vi "Read initial setup.vi"(8 "error in (no error)":errorcluster, 10 "use cong file":bool, 11 "Channel in":refnum<class "SPARC4_Channel.lvclass">) -> (0 "error out":errorcluster, 3 "Channel out":refnum<class "SPARC4_Channel.lvclass">)   [LabVIEW 2018, in "SPARC4_Channel.lvclass"]
uses:
  SPARC4_Channel.lvclass
  SPARC4_Channel.lvclass/SPARC4_Channel.ctl
  <vilib>/Utility/config.llb/Read Key (U32).vi
  <vilib>/Utility/config.llb/Read Key (String).vi
  <vilib>/Utility/config.llb/NI_LVConfig.lvlib
panel:
  out "Configuration to initialize ACS":T1
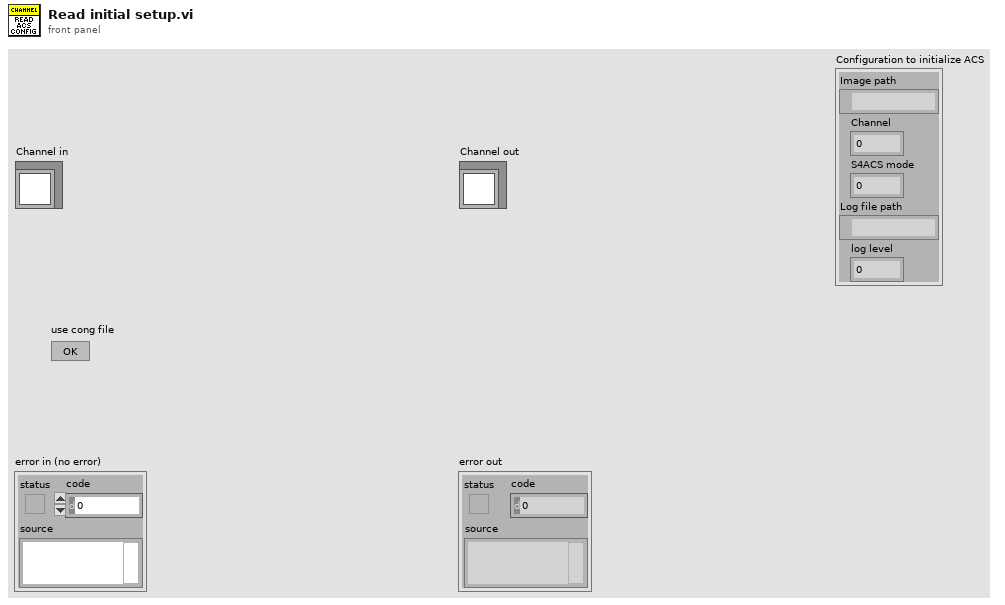
[diagram p1: front panel]
types:
  T1 = cluster{"Image path":path, "Channel":u8, "S4ACS mode":u16, "Log file path":path, "log level":u16}
  T2 = typedef "NI_LVConfig.lvlib/Config Data RefNum.ctl" = refnum<k1>
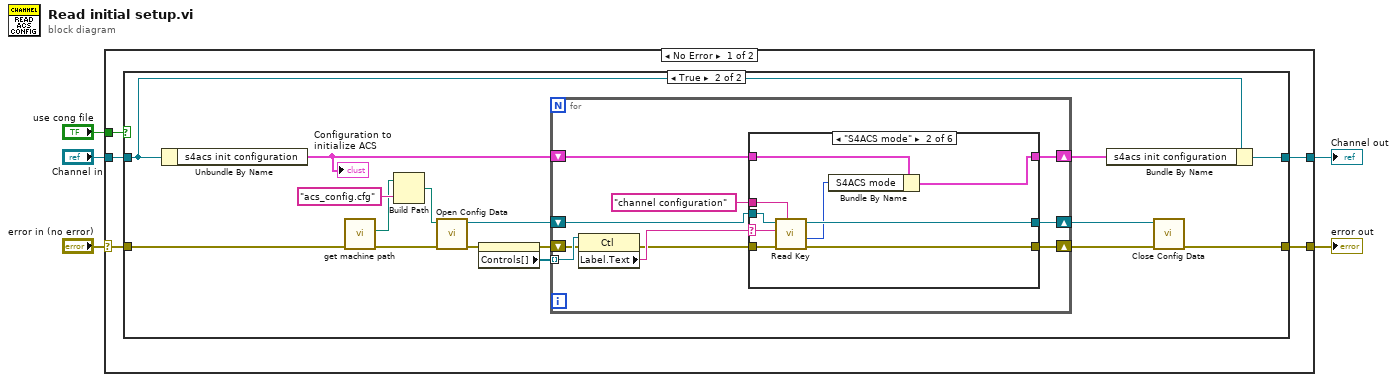
[diagram p0: block diagram]
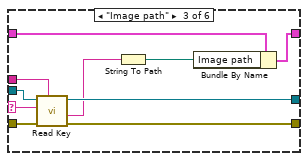
[diagram p4: hidden frame]
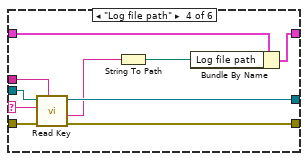
[diagram p5: hidden frame]
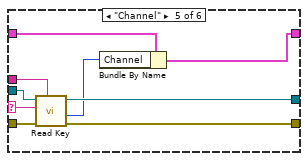
[diagram p6: hidden frame]
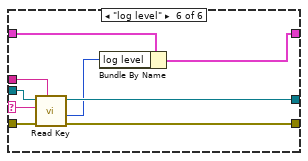
[diagram p7: hidden frame]
diagram:
  n1 = case shown="No Error" "error in (no error)" {
    selector: "error in (no error)" -> [w7 w90]
    tunnel: [w10 w90] -> w3
    tunnel: [w8 w89] -> w2
    tunnel: "Channel in" -> [w9 w89]
    tunnel: "use cong file" -> [w6 _]
    frame No Error {
      n2 = case shown="True" w6 {
        tunnel: [w11 w25] -> w10
        tunnel: w9 -> [w12 w24]
        tunnel: [w12 w22] -> w8
        tunnel: w7 -> [w11 w18]
        frame False {
        }
        frame True {
          n3 = Unbundle By Name(w24) -> ("s4acs init configuration"=w16:T1)
          "Configuration to initialize ACS" <- w16
          n4 = call "get machine path.vi"("error in (no error) 2"=w18) -> ("error in (no error)"=w19:errorcluster, "machine path"=w17:path)  [unwired: 9 in]
          n5 = Build Path(base path=w17, name or relative path="acs_config.cfg") -> (appended path=w21:path)
          n6 = call <vilib>:"Open Config Data.vi"("error in (no error)"=w19, "configuration file path"=w21) -> ("error out"=w13:errorcluster, "refnum"=w27:T2)  [unwired: 7 in, 1 out]
          n7 = property on="Configuration to initialize ACS" class="Clust (strict)"(error in=w13) -> (error out=w14:errorcluster, "Controls[]"=w15:refnum<vi>[])  [unwired: 1 in, 1 out]
          n8 = for {
            tunnel: w15 -> [w37] mode=indexing
            shift-right: [w35] -> w28
            shift-left: w14 -> [w33]
            shift-right: [w34] -> w26
            shift-left: w27 -> [w32]
            shift-right: [w30] -> w23
            shift-left: w16 -> [w38]
            n9 = property class="Ctl"(reference=w37, error in=w33) -> (error out=w31:errorcluster, "Label.Text"=w36:string)  [unwired: 1 out]
            n10 = case shown="\"S4ACS mode\"" w36 {
              selector: w36 -> [_ w48 w58 w68 w77 w86]
              tunnel: [w40 w49 w59 w69 w78 w87] -> w34
              tunnel: [w39 w50 w60 w70 w79 w88] -> w35
              tunnel: w38 -> [w41 w46 w55 w65 w75 w84]
              tunnel: [w41 w45 w54 w64 w74 w83] -> w30
              tunnel: w32 -> [w40 w43 w52 w62 w73 w82]
              tunnel: w31 -> [w39 w42 w51 w61 w72 w81]
              tunnel: "channel configuration" -> [_ w44 w53 w63 w71 w80]
              frame "False", Default {
              }
              frame "S4ACS mode" {
                n11 = call-poly <vilib>:"Read Key.vi"("section"=w44, "error in (no error)"=w42, "key"=w48, "refnum"=w43) -> ("error out"=w50:errorcluster, "value"=w47:u32, "refnum out"=w49:T2)  [unwired: 4 in, 1 out]
                n12 = Bundle By Name(cluster=w46, "S4ACS mode"=w47) -> (w45:T1)
              }
              frame "Image path" {
                n13 = call-poly <vilib>:"Read Key.vi"("section"=w53, "error in (no error)"=w51, "key"=w58, "refnum"=w52) -> ("error out"=w60:errorcluster, "value"=w56:string, "refnum out"=w59:T2)  [unwired: 4 in, 1 out]
                n14 = String To Path(string=w56) -> (path=w57:path)
                n15 = Bundle By Name(cluster=w55, "Image path"=w57) -> (w54:T1)
              }
              frame "Log file path" {
                n16 = call-poly <vilib>:"Read Key.vi"("section"=w63, "error in (no error)"=w61, "key"=w68, "refnum"=w62) -> ("error out"=w70:errorcluster, "value"=w66:string, "refnum out"=w69:T2)  [unwired: 4 in, 1 out]
                n17 = String To Path(string=w66) -> (path=w67:path)
                n18 = Bundle By Name(cluster=w65, "Log file path"=w67) -> (w64:T1)
              }
              frame "Channel" {
                n19 = call-poly <vilib>:"Read Key.vi"("section"=w71, "error in (no error)"=w72, "key"=w77, "refnum"=w73) -> ("error out"=w79:errorcluster, "value"=w76:u32, "refnum out"=w78:T2)  [unwired: 4 in, 1 out]
                n20 = Bundle By Name(cluster=w75, "Channel"=w76) -> (w74:T1)
              }
              frame "log level" {
                n21 = call-poly <vilib>:"Read Key.vi"("section"=w80, "error in (no error)"=w81, "key"=w86, "refnum"=w82) -> ("error out"=w88:errorcluster, "value"=w85:u32, "refnum out"=w87:T2)  [unwired: 4 in, 1 out]
                n22 = Bundle By Name(cluster=w84, "log level"=w85) -> (w83:T1)
              }
            }
          }
          n23 = Bundle By Name(cluster=w24, "s4acs init configuration"=w23) -> (w22:refnum<class "SPARC4_Channel.lvclass">)
          n24 = call <vilib>:"Close Config Data.vi"("error in (no error)"=w28, "refnum"=w26) -> ("error out"=w25:errorcluster)  [unwired: 8 in, 1 out]
        }
      }
    }
    frame Error {
    }
  }
  "error out" <- w3
  "Channel out" <- w2
